vi "uEye_Eeprom.vi"() -> ()   [LabVIEW 2010]
uses:
  C:/Program Files (x86)/National Instruments/LabVIEW 2016/instr.lib/IDS/ueye.NET/uEyeDotNet.dll
  Program Files (x86)/National Instruments/LabVIEW 2016/instr.lib/IDS/ueye.NET/uEyeDotNet.dll
panel:
  in  "Text":string
  in  "Write 3":bool
  out "Read":string
  out "Image":picture
  in  "Camera ID":i32 min=0 max=255
  out "Serial Number":string
  out "AOI Height":i32=8
  out "AOI Width":i32=8
  out "Bits/Pixel":i32=8
  out "Error Out":errorcluster caption="error"
  in  "Exit Camera":bool
  in  "Init Camera":bool
  # "EEPROM"
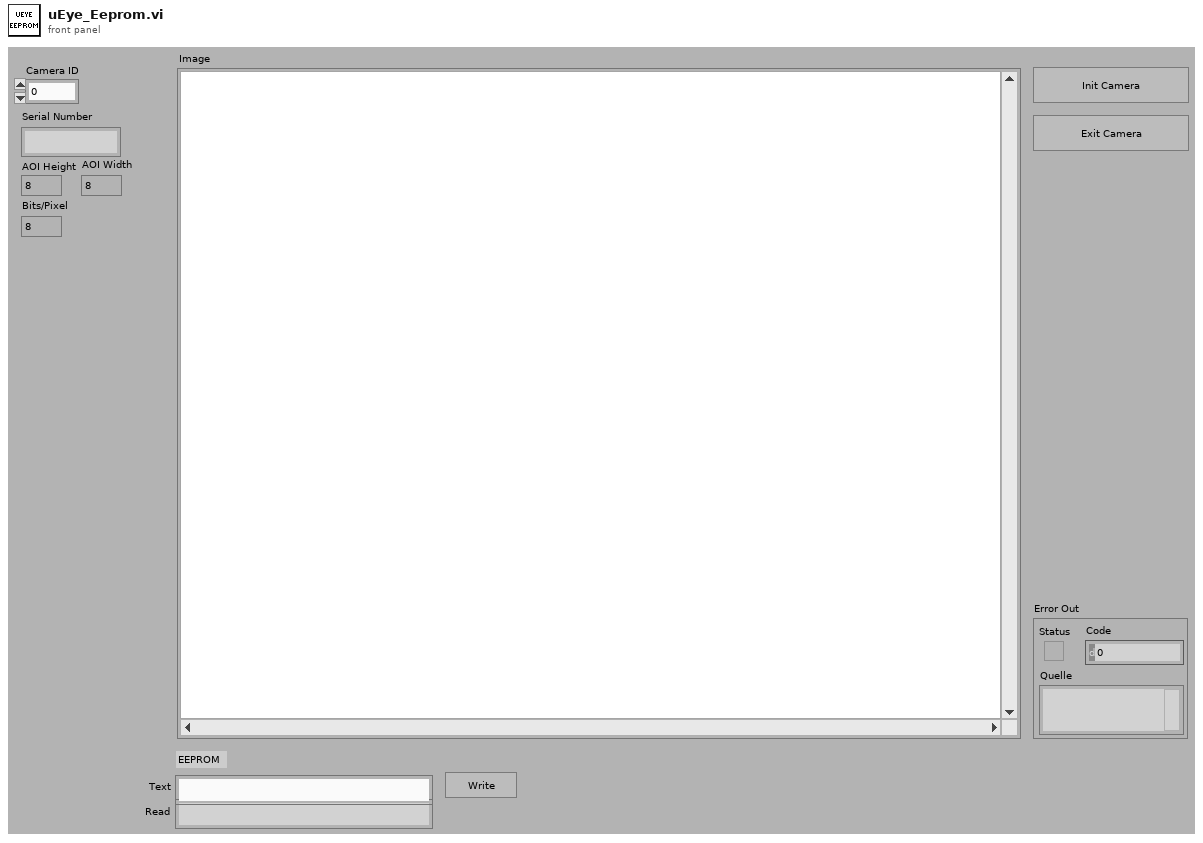
[diagram p1: front panel]
types:
  T1 = enum8{"Enabled", "Disabled", "Disabled and Grayed Out"}
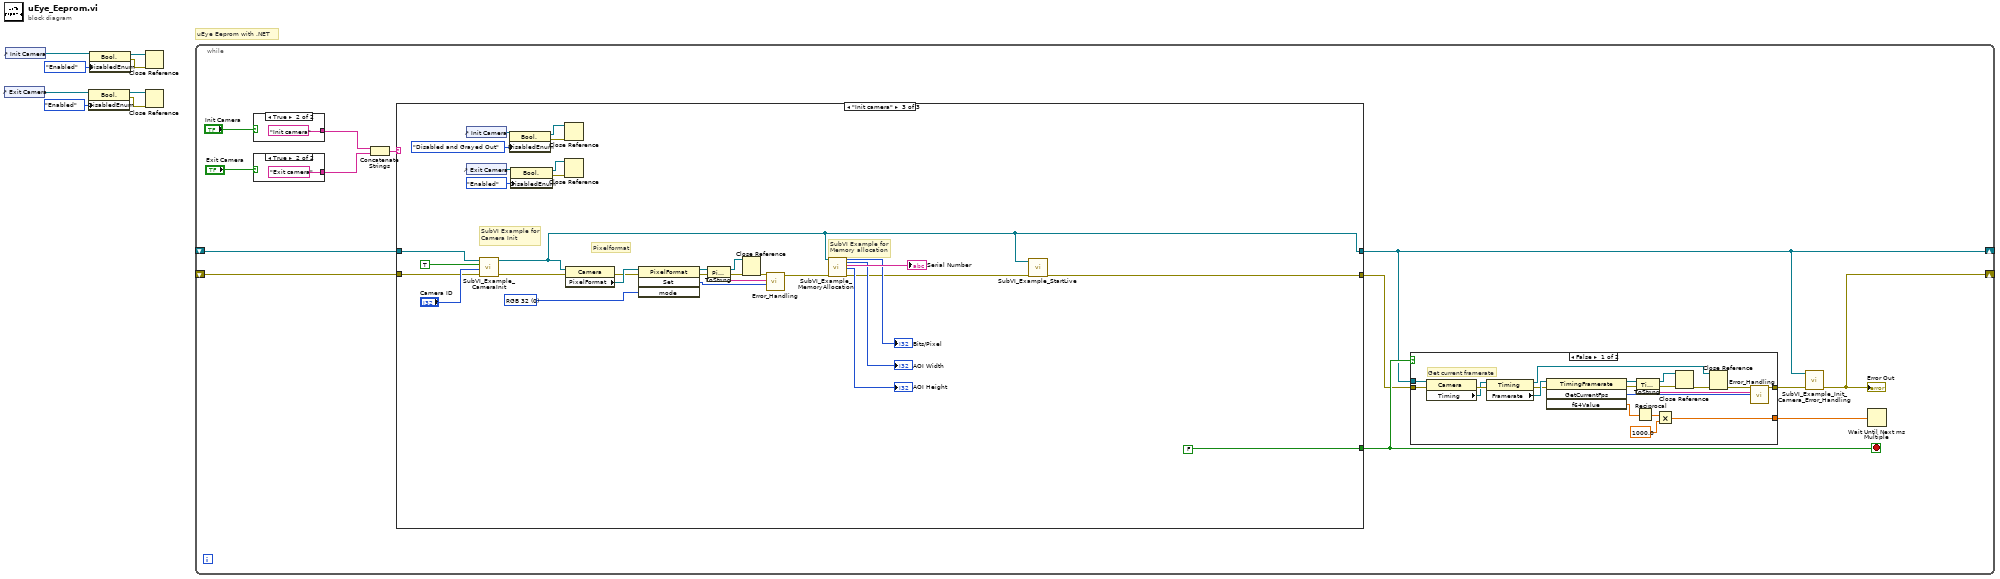
[diagram p0: block diagram]
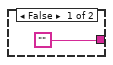
[diagram p2: hidden frame]
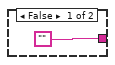
[diagram p3: hidden frame]
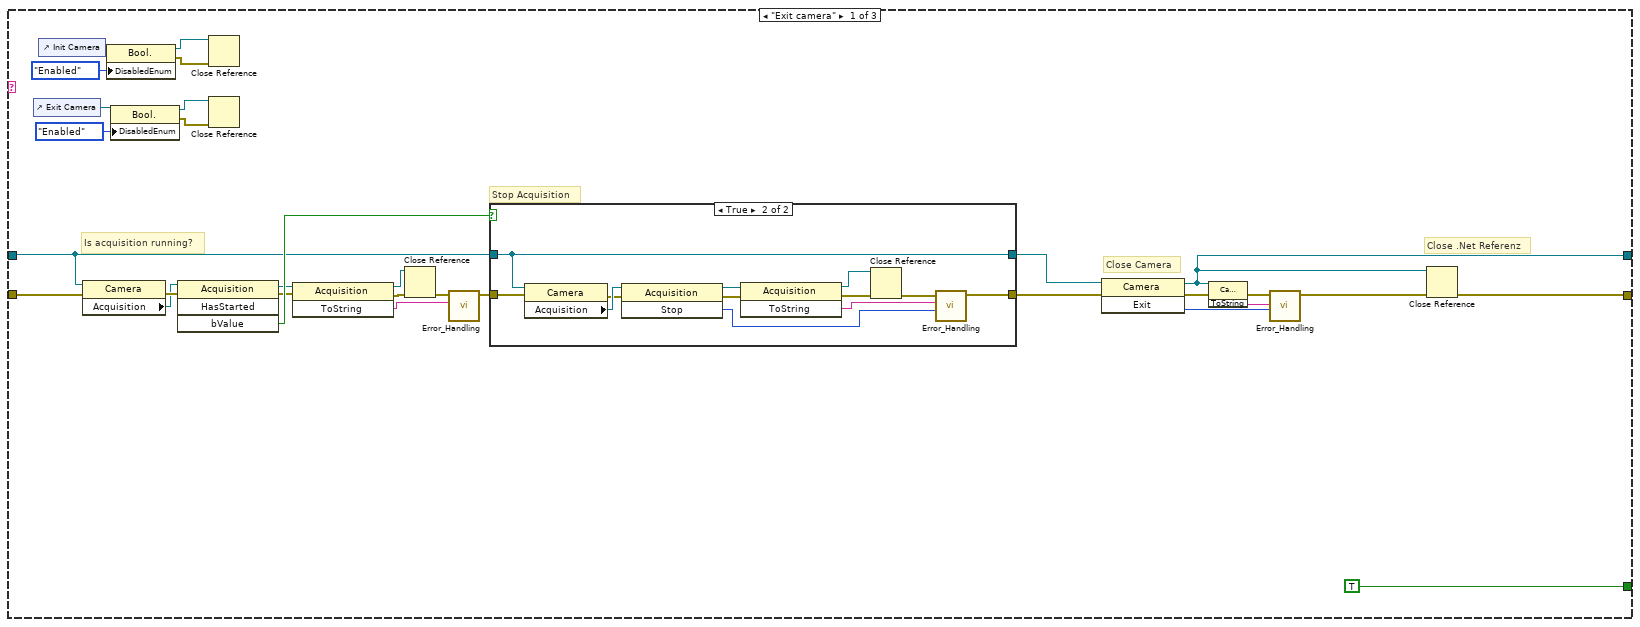
[diagram p4: hidden frame]
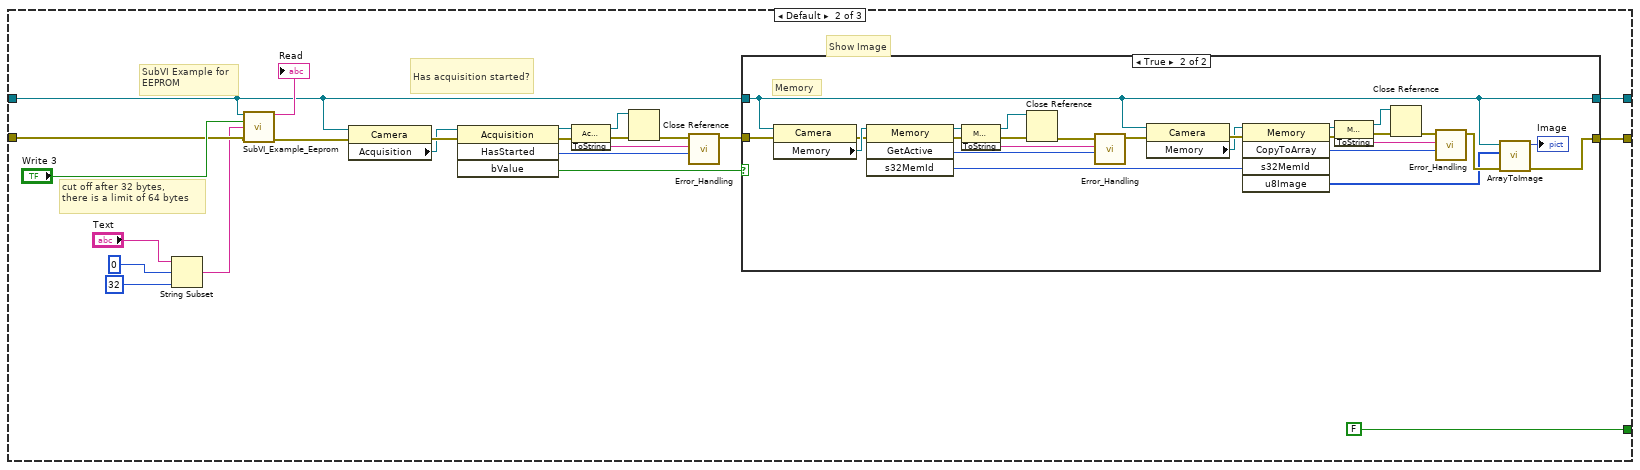
[diagram p6: hidden frame]
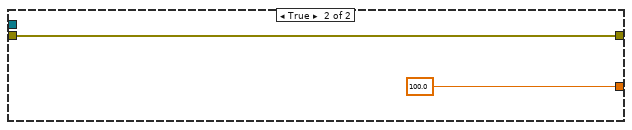
[diagram p8: hidden frame]
diagram:
  # "uEye Eeprom with .NET"
  n1 = control-ref of="Exit Camera"() -> (w5:refnum<vi>)
  n2 = control-ref of="Init Camera"() -> (w7:refnum<vi>)
  n3 = property class="Bool."(reference=w5, "DisabledEnum"=T1."Enabled" ("Disabled")) -> (reference out=w1:refnum<vi>, error out=w2:errorcluster)  [unwired: 1 in]
  n4 = property class="Bool."(reference=w7, "DisabledEnum"=T1."Enabled" ("Disabled")) -> (reference out=w4:refnum<vi>, error out=w3:errorcluster)  [unwired: 1 in]
  n5 = Close Reference(reference=w4, error in (no error)=w3) -> ()  [unwired: 1 out]
  n6 = Close Reference(reference=w1, error in (no error)=w2) -> ()  [unwired: 1 out]
  n7 = while {
    shift-right: [w10] -> _
    shift-left: _ -> [w14]
    shift-right: [w9] -> _
    shift-left: _ -> [w15]
    stop <- w13 stop-if-true
    n8 = case shown="True" "Init Camera" {
      tunnel: ["" "Init camera"] -> w19
      frame False {
      }
      frame True {
      }
    }
    n9 = case shown="True" "Exit Camera" {
      tunnel: ["" "Exit camera"] -> w16
      frame False {
      }
      frame True {
      }
    }
    n10 = Concatenate Strings(w19, w16) -> (w18:string)
    n11 = case shown="\"Init camera\"" w18 {
      tunnel: w15 -> [w40 w78 w144]
      tunnel: w14 -> [w39 w77 w143]
      tunnel: [w38 w83 w132] -> w9
      tunnel: [w37 w82 w133] -> w12
      tunnel: [TRUE FALSE FALSE] -> w13
      frame "Exit camera" {
        # "Close .Net Referenz"
        # "Is acquisition running?"
        # "Stop Acquisition"
        # "Close Camera"
        n12 = control-ref of="Exit Camera"() -> (w33:refnum<vi>)
        n13 = control-ref of="Init Camera"() -> (w34:refnum<vi>)
        n14 = property class="Camera"(reference=w40, error in=w39) -> (error out=w49:errorcluster, "Acquisition"=w48:refnum<k24>)  [unwired: 1 out]
        n15 = property class="Bool."(reference=w34, "DisabledEnum"=T1."Enabled" ("Disabled")) -> (reference out=w29:refnum<vi>, error out=w28:errorcluster)  [unwired: 1 in]
        n16 = property class="Bool."(reference=w33, "DisabledEnum"=T1."Enabled" ("Disabled")) -> (reference out=w27:refnum<vi>, error out=w26:errorcluster)  [unwired: 1 in]
        n17 = invoke class="Acquisition" method="HasStarted"(reference=w48, error in=w49) -> (reference out=w43:refnum<k24>, error out=w45:errorcluster, "bValue"=w47:bool)  [unwired: 2 in, 1 out]
        n18 = Close Reference(reference=w29, error in (no error)=w28) -> ()  [unwired: 1 out]
        n19 = Close Reference(reference=w27, error in (no error)=w26) -> ()  [unwired: 1 out]
        n20 = invoke class="Acquisition" method="ToString"(reference=w43, error in=w45) -> (reference out=w30:refnum<k24>, error out=w32:errorcluster, "ToString"=w44:string)  [unwired: 1 in]
        n21 = Close Reference(reference=w30, error in (no error)=w32) -> (error out=w31:errorcluster)
        n22 = call "Error_Handling.vi"("Error String"=w44, "Error In"=w31) -> ("Error Out"=w46:errorcluster)  [unwired: 9 in]
        n23 = case shown="True" w47 {
          tunnel: [w57 w68] -> w41
          tunnel: w46 -> [w57 w69]
          tunnel: w40 -> [w56 w61]
          tunnel: [w56 w61] -> w42
          frame False {
          }
          frame True {
            n24 = property class="Camera"(reference=w61, error in=w69) -> (error out=w65:errorcluster, "Acquisition"=w66:refnum<k24>)  [unwired: 1 out]
            n25 = invoke class="Acquisition" method="Stop"(reference=w66, error in=w65) -> (reference out=w63:refnum<k24>, error out=w64:errorcluster, "Stop"=w62:i32)  [unwired: 1 in]
            n26 = invoke class="Acquisition" method="ToString"(reference=w63, error in=w64) -> (reference out=w58:refnum<k24>, error out=w60:errorcluster, "ToString"=w67:string)  [unwired: 1 in]
            n27 = Close Reference(reference=w58, error in (no error)=w60) -> (error out=w59:errorcluster)
            n28 = call "Error_Handling.vi"("Error Code"=w62, "Error String"=w67, "Error In"=w59) -> ("Error Out"=w68:errorcluster)  [unwired: 8 in]
          }
        }
        n29 = invoke class="Camera" method="Exit"(reference=w42, error in=w41) -> (reference out=w38:refnum<k24>, error out=w52:errorcluster, "Exit"=w51:i32)  [unwired: 1 in]
        n30 = invoke class="Camera" method="ToString"(reference=w38, error in=w52) -> (error out=w53:errorcluster, "ToString"=w54:string)  [unwired: 1 in, 1 out]
        n31 = call "Error_Handling.vi"("Error Code"=w51, "Error String"=w54, "Error In"=w53) -> ("Error Out"=w50:errorcluster)  [unwired: 8 in]
        n32 = Close Reference ("Close Referenz")(reference=w38, error in (no error)=w50) -> (error out=w37:errorcluster)
      }
      frame Default {
        # "cut off after 32 bytes,\nthere is a limit of 64 bytes"
        # "SubVI Example for\nEEPROM"
        # "Has acquisition started?"
        # "Show Image"
        n33 = String Subset(string="Text", offset (0)=0, length (rest)=32 ("length (rest)")) -> (substring=w73:string)
        n34 = call "SubVI_Example_Eeprom.vi"(".NET (Reference)"=w78, "Write Flag"="Write 3", "Input Data"=w73, "Error In"=w77) -> ("Eeprom Data"=→"Read":string, "Error Out"=w81:errorcluster)  [unwired: 10 in]
        n35 = property class="Camera"(reference=w78, error in=w81) -> (error out=w91:errorcluster, "Acquisition"=w90:refnum<k24>)  [unwired: 1 out]
        n36 = invoke class="Acquisition" method="HasStarted"(reference=w90, error in=w91) -> (reference out=w87:refnum<k24>, error out=w86:errorcluster, "HasStarted"=w85:i32, "bValue"=w89:bool)  [unwired: 2 in]
        n37 = invoke class="Acquisition" method="ToString"(reference=w87, error in=w86) -> (reference out=w70:refnum<k24>, error out=w72:errorcluster, "ToString"=w88:string)  [unwired: 1 in]
        n38 = Close Reference(reference=w70, error in (no error)=w72) -> (error out=w71:errorcluster)
        n39 = call "Error_Handling.vi"("Error Code"=w85, "Error String"=w88, "Error In"=w71) -> ("Error Out"=w84:errorcluster)  [unwired: 8 in]
        n40 = case shown="True" w89 {
          tunnel: [w94 w106] -> w82
          tunnel: w84 -> [w94 w105]
          tunnel: w78 -> [w93 w102]
          tunnel: [w93 w102] -> w83
          frame False {
          }
          frame True {
            # "Memory"
            n41 = property class="Camera"(reference=w102, error in=w105) -> (error out=w108:errorcluster, "Memory"=w109:refnum<k24>)  [unwired: 1 out]
            n42 = invoke class="Memory" method="GetActive"(reference=w109, error in=w108) -> (reference out=w114:refnum<k24>, error out=w113:errorcluster, "GetActive"=w115:i32, "s32MemId"=w107:i32)  [unwired: 2 in]
            n43 = invoke class="Memory" method="ToString"(reference=w114, error in=w113) -> (reference out=w95:refnum<k24>, error out=w97:errorcluster, "ToString"=w112:string)  [unwired: 1 in]
            n44 = Close Reference(reference=w95, error in (no error)=w97) -> (error out=w96:errorcluster)
            n45 = call "Error_Handling.vi"("Error Code"=w115, "Error String"=w112, "Error In"=w96) -> ("Error Out"=w116:errorcluster)  [unwired: 8 in]
            n46 = property class="Camera"(reference=w102, error in=w116) -> (error out=w111:errorcluster, "Memory"=w110:refnum<k24>)  [unwired: 1 out]
            n47 = invoke class="Memory" method="CopyToArray"(reference=w110, error in=w111, "s32MemId"=w107) -> (reference out=w118:refnum<k24>, error out=w119:errorcluster, "CopyToArray"=w120:i32, "u8Image"=w103:u8[])  [unwired: 2 in, 1 out]
            n48 = invoke class="Memory" method="ToString"(reference=w118, error in=w119) -> (reference out=w98:refnum<k24>, error out=w100:errorcluster, "ToString"=w117:string)  [unwired: 1 in]
            n49 = Close Reference(reference=w98, error in (no error)=w100) -> (error out=w99:errorcluster)
            n50 = call "Error_Handling.vi"("Error Code"=w120, "Error String"=w117, "Error In"=w99) -> ("Error Out"=w104:errorcluster)  [unwired: 8 in]
            n51 = call "ArrayToImage.vi"("Error In"=w104, "InArray"=w103, ".NET (Reference)"=w102) -> ("Error Out"=w106:errorcluster, "Image"=→"Image":picture)  [unwired: 7 in]
          }
        }
      }
      frame "Init camera" {
        w152 = 0 items=["RGB 32"=0, "RGB 24"=1, "Y8 Monochrom"=6] ("Mode")
        # "SubVI Example for \nMemory allocation"
        # "SubVI Example for \nCamera Init"
        # "Pixelformat"
        n52 = control-ref of="Init Camera"() -> (w130:refnum<vi>)
        n53 = control-ref of="Exit Camera"() -> (w128:refnum<vi>)
        n54 = call "SubVI_Example_CameraInit.vi"("Error In"=w143, "Camera ID"="Camera ID", "Init Camera Flag"=TRUE, ".NET (Reference)"=w144) -> ("Error Out"=w149:errorcluster, ".NET (Reference)"=w132:refnum<k24>)  [unwired: 6 in]
        n55 = property class="Bool."(reference=w130, "DisabledEnum"=T1."Disabled and Grayed Out" ("Disabled")) -> (reference out=w124:refnum<vi>, error out=w123:errorcluster)  [unwired: 1 in]
        n56 = property class="Bool."(reference=w128, "DisabledEnum"=T1."Enabled" ("Disabled")) -> (reference out=w122:refnum<vi>, error out=w121:errorcluster)  [unwired: 1 in]
        n57 = Close Reference(reference=w124, error in (no error)=w123) -> ()  [unwired: 1 out]
        n58 = Close Reference(reference=w122, error in (no error)=w121) -> ()  [unwired: 1 out]
        n59 = property on="Property Node" class="Camera"(reference=w132, error in=w149) -> (error out=w150:errorcluster, "PixelFormat"=w151:refnum<k24>)  [unwired: 1 out]
        n60 = invoke class="PixelFormat" method="Set"(reference=w151, error in=w150, "mode"=w152) -> (reference out=w147:refnum<k24>, error out=w140:errorcluster, "Set"=w146:i32)  [unwired: 1 in, 1 out]
        n61 = invoke class="PixelFormat" method="ToString"(reference=w147, error in=w140) -> (reference out=w125:refnum<k24>, error out=w127:errorcluster, "ToString"=w148:string)  [unwired: 1 in]
        n62 = Close Reference(reference=w125, error in (no error)=w127) -> (error out=w126:errorcluster)
        n63 = call "Error_Handling.vi"("Error Code"=w146, "Error String"=w148, "Error In"=w126) -> ("Error Out"=w135:errorcluster)  [unwired: 8 in]
        n64 = call "SubVI_Example_MemoryAllocation.vi"(".NET (Reference)"=w132, "Error In"=w135) -> ("Bits/Pixel 2"=→"Bits/Pixel":i32, "Width"=→"AOI Width":i32, "Serial Number"=→"Serial Number":string, "Height"=→"AOI Height":i32, "Error Out"=w134:errorcluster)  [unwired: 13 in]
        n65 = call "SubVI_Example_StartLive.vi"("Error"=w134, ".NET (Reference)"=w132) -> ("Error"=w133:errorcluster)  [unwired: 9 in]
      }
    }
    n66 = case shown="False" w13 {
      tunnel: [w165 100.0] -> w21
      tunnel: w9 -> [w164 _]
      tunnel: w12 -> [w163 w174]
      tunnel: [w160 w174] -> w11
      frame False {
        # "Get current framerate"
        n67 = property class="Camera"(reference=w164, error in=w163) -> (error out=w167:errorcluster, "Timing"=w166:refnum<k24>)  [unwired: 1 out]
        n68 = property class="Timing"(reference=w166, error in=w167) -> (reference out=w153:refnum<k24>, error out=w169:errorcluster, "Framerate"=w170:refnum<k24>)
        n69 = invoke class="TimingFramerate" method="GetCurrentFps"(reference=w170, error in=w169) -> (reference out=w158:refnum<k24>, error out=w159:errorcluster, "GetCurrentFps"=w161:i32, "f64Value"=w168:dbl)  [unwired: 2 in]
        n70 = Reciprocal(x=w168) -> (1/x=w172:dbl)
        n71 = invoke class="TimingFramerate" method="ToString"(reference=w158, error in=w159) -> (reference out=w154:refnum<k24>, error out=w157:errorcluster, "ToString"=w162:string)  [unwired: 1 in]
        n72 = Multiply(x=w172, y=1000.0) -> (x*y=w165:dbl)
        n73 = Close Reference(reference=w154, error in (no error)=w157) -> (error out=w156:errorcluster)
        n74 = Close Reference(reference=w153, error in (no error)=w156) -> (error out=w155:errorcluster)
        n75 = call "Error_Handling.vi"("Error Code"=w161, "Error String"=w162, "Error In"=w155) -> ("Error Out"=w160:errorcluster)  [unwired: 8 in]
      }
      frame True {
      }
    }
    n76 = call "SubVI_Example_Init_Camera_Error_Handling.vi"("Error In"=w11, ".NET (Reference)"=w9) -> ("Error Out"=w10:errorcluster)  [unwired: 9 in]
    "Error Out" <- w10
    n77 = Wait Until Next ms Multiple(millisecond multiple=w21) -> ()  [unwired: 1 out]
  }
